vi "Replace Regexp String.vi"(1 "Search String":string="\\n", 2 "Input String":string="This is a test\nit is a real test\nlet's see what is in\nthis box?\ntesting?\n", 3 "Replacement String":string="\r") -> (0 "Output String":string="This is a test\rit is a real test\rlet's see what is in\rthis box?\rtesting?\r")   [LabVIEW 2019]
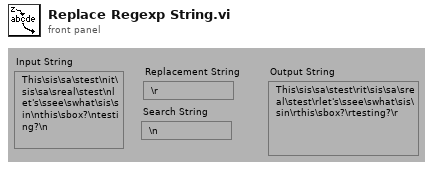
[diagram p1: front panel]
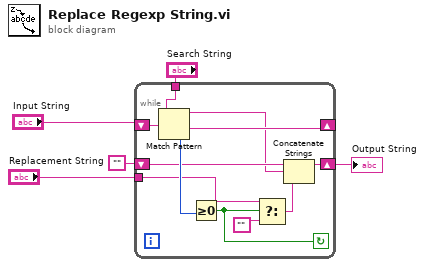
[diagram p0: block diagram]
diagram:
  n1 = while {
    tunnel: "Replacement String" -> [w8]
    shift-left: "Input String" -> [w14]
    shift-right: [w13] -> _
    shift-left: "" -> [w12]
    shift-right: [w11] -> w1
    tunnel: "Search String" -> [w16]
    stop <- w9 continue-if-true
    n2 = Match Pattern(string=w14, regular expression=w16) -> (before substring=w10:string, after substring=w13:string, offset past match=w15:i32)  [unwired: 1 in, 1 out]
    n3 = Greater Or Equal To 0?(x=w15) -> (x >= 0?=w9:bool)
    n4 = Select(t=w8, s=w9, f="") -> (s? t:f=w7:string)
    n5 = Concatenate Strings(w12, w10, w7) -> (w11:string)
  }
  "Output String" <- w1
